vi "absCalcPlot_III.vi"(5 "file path (dialog if empty)":path, 6 "Cell Calibration, mV/mW":dbl=600000.0, 7 "save?":bool, 8 "Error In":errorcluster, 9 "PD Values":cluster{dbl, dbl, dbl}, 10 "bkg values":cluster{dbl, dbl, dbl}, 11 "Mic Values":cluster{dbl, dbl, dbl}) -> (0 "Error Out":errorcluster, 1 "aae":dbl, 2 "Time Series":cluster{dbl, dbl, dbl}, 3 "Spectrum":cluster{dbl[], "Best Power Fit":dbl[]}[](graph))   [LabVIEW 2011]
uses:
  saveTimeSeries_III.vi
  <vilib>/Analysis/NI_AALPro.lvlib
panel:
  out "output cluster":cluster{i32[], "Best Power Fit":dbl[]}
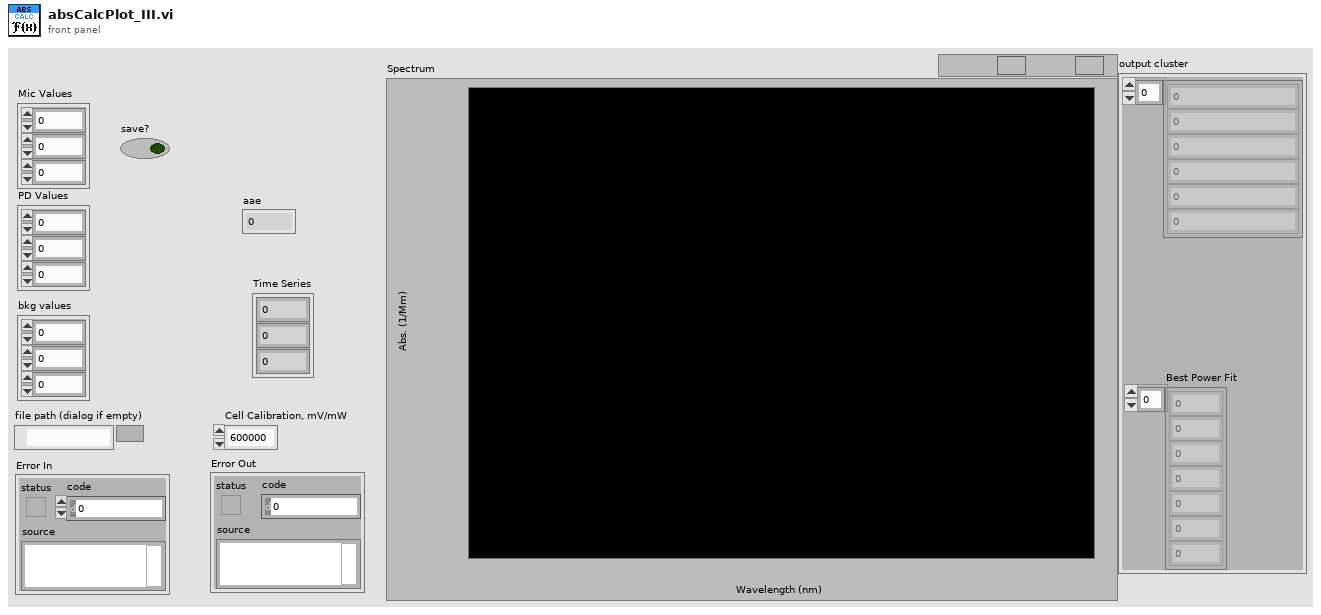
[diagram p1: front panel]
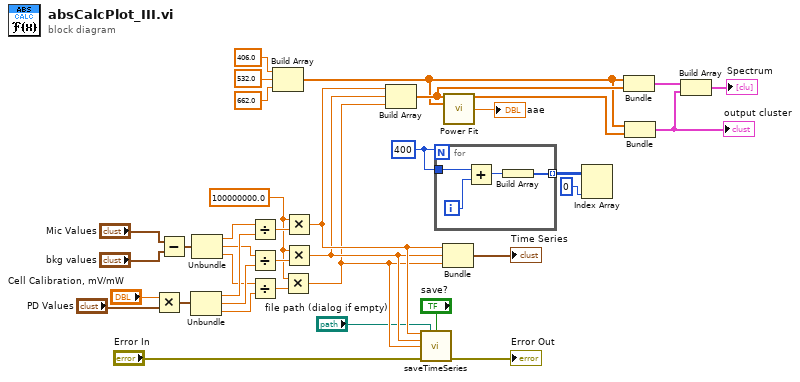
[diagram p0: block diagram]
diagram:
  w12 = 100000000.0 ("element")
  w21 = 400
  n1 = Multiply(x="Cell Calibration, mV/mW", y="PD Values") -> (x*y=w31:cluster{dbl, dbl, dbl})
  n2 = Subtract(x="Mic Values", y="bkg values") -> (x-y=w23:cluster{dbl, dbl, dbl})
  n3 = Unbundle(w31) -> (w32:dbl, w33:dbl, w34:dbl)
  n4 = Unbundle(w23) -> (w26:dbl, w27:dbl, w28:dbl)
  n5 = Divide(x=w26, y=w32) -> (x/y=w15:dbl)
  n6 = Divide(x=w27, y=w33) -> (x/y=w14:dbl)
  n7 = Divide(x=w28, y=w34) -> (x/y=w13:dbl)
  n8 = Build Array(406.0 ("element"), 532.0 ("element"), 662.0 ("element")) -> (w9:dbl[])
  n9 = Multiply(x=w12, y=w13) -> (x*y=w3:dbl)
  n10 = Multiply(x=w12, y=w15) -> (x*y=w5:dbl)
  n11 = Multiply(x=w12, y=w14) -> (x*y=w4:dbl)
  n12 = Build Array(w5, w4, w3) -> (w10:dbl[])
  n13 = call-poly "saveTimeSeries.vi"("422nm"=w5, "file path (dialog if empty)"="file path (dialog if empty)", "save?"="save?", "532nm"=w4, "785nm"=w3, "Error In"="Error In") -> ("Error Out"=→"Error Out":errorcluster)  [unwired: 9 in]
  n14 = for {
    N: w21 -> [_]
    tunnel: w21 -> [w40]
    tunnel: [w38] -> w19 mode=indexing
    i -> [w41]
    n15 = Add(x=w40, y=w41) -> (x+y=w39:i32)
    n16 = Build Array(w39) -> (w38:i32[])
  }
  n17 = Bundle(w5, w4, w3) -> (→"Time Series":cluster{dbl, dbl, dbl})  [unwired: 1 in]
  n18 = call <vilib>:"Power Fit.vi"("Y"=w10, "X"=w9) -> ("Best Power Fit"=w20:dbl[], "power"=→"aae":dbl)  [unwired: 8 in, 4 out]
  n19 = Index Array(array=w19, index (col)=0 ("index (row)")) -> ()  [unwired: 1 in, 1 out]
  n20 = Bundle(w9, w10) -> (w8:cluster{dbl[], dbl[]})  [unwired: 1 in]
  n21 = Bundle(w9, "Best Power Fit"=w20) -> (w18:cluster{dbl[], "Best Power Fit":dbl[]})  [unwired: 1 in]
  "output cluster" <- w18
  n22 = Build Array(w8, w18) -> (→"Spectrum":cluster{dbl[], "Best Power Fit":dbl[]}[])
